vi "Exit.vi"(8 "error in":errorcluster) -> (0 "error out":errorcluster)   [LabVIEW 2018, in "Controller (Host).lvlib"]
doc: "This subVI enqueues the named action in to the communications queue along with the input data."
uses:
  Controller (Host).lvlib
  Private Controls/Module Data.ctl
  Private Controls/Module Action.ctl
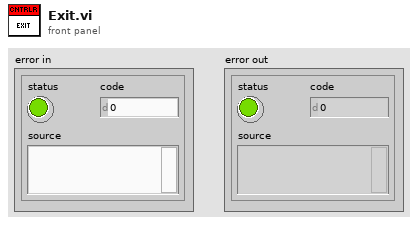
[diagram p1: front panel]
types:
  T1 = typedef "Controller (Host).lvlib/Module Data.ctl" = cluster{"Data":variant, "Action":T2}
  T2 = typedef "Controller (Host).lvlib/Module Action.ctl" = enum8{"Timeout", "New Data", "Value to Monitor", "Init", "Reset Dev_Min_Max", "Error", "Exit", "Prompt Test Info", "Update Test Info", "Prompt Variable Info", "Load APU Setup Data"}
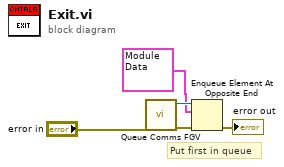
[diagram p0: block diagram]
diagram:
  # "Put first in queue"
  n1 = call "Queue Comms FGV.vi"("error in (no error)"="error in") -> ("error out"=w3:errorcluster, "Queue out"=w2:refnum<queue>)  [unwired: 9 in]
  n2 = Enqueue Element At Opposite End(queue=w2, element=T1 {"Data"=variant, "Action"=enum."Exit"}, error in (no error)=w3) -> (error out=→"error out":errorcluster)  [unwired: 1 in, 2 out]
